vi "Initialize Picture Drag.vi"(6 "wheel index":i32, 8 "error in (no error)":errorcluster, 9 "dragging mode":T1, 10 "global mouse position":cluster{"x":dbl, "y":dbl}, 11 "dialog info in":T2={"steering frame ref"=refnum, "active wheel indexes"=[], "FP Refs"={"VI Refnum"=refnum, "Menu Ref"=refnum, "Sub Panel"=refnum, "picture"=refnum, "Steering Type"=refnum, "zoom in"=refnum, "zoom out"=refnum, "zoom extents"=refnum, "Wheels"=refnum, "Add Wheel"=refnum, "Remove Wheel"=refnum, "Copy Wheel"=refnum, "Angle Units"=refnum}, "subpanel info"={"subpanel VI refs"=[], "subpanel types"=[], "main to subpanel command events"=[]}, "picture dragging state"={"dragging"=FALSE, "wheel index"=-1, "dragging mode"=enum."translate", "wheel start position"={"x"=0.0, "y"=0.0, "theta"=0.0}, "relative mouse position"={"x"=0.0, "y"=0.0}, "relative mouse init angle (rad)"=0.0}, "picture size (pixels)"={"Width"=500, "Height"=500}, "picture grid"=bytes[0], "click zones group"={"click zones array"=[], "num click zones"=0}, "draw options"={"draw wheel states?"=FALSE, "highlight wheel index"=-1, "pixels per unit"=10.0, "draw forward velocity?"=FALSE, "velocity scale"=1.0}}) -> (0 "error out":errorcluster, 3 "dialog info out":T2={"steering frame ref"=refnum, "active wheel indexes"=[], "FP Refs"={"VI Refnum"=refnum, "Menu Ref"=refnum, "Sub Panel"=refnum, "picture"=refnum, "Steering Type"=refnum, "zoom in"=refnum, "zoom out"=refnum, "zoom extents"=refnum, "Wheels"=refnum, "Add Wheel"=refnum, "Remove Wheel"=refnum, "Copy Wheel"=refnum, "Angle Units"=refnum}, "subpanel info"={"subpanel VI refs"=[], "subpanel types"=[], "main to subpanel command events"=[]}, "picture dragging state"={"dragging"=FALSE, "wheel index"=-1, "dragging mode"=enum."translate", "wheel start position"={"x"=0.0, "y"=0.0, "theta"=0.0}, "relative mouse position"={"x"=0.0, "y"=0.0}, "relative mouse init angle (rad)"=0.0}, "picture size (pixels)"={"Width"=500, "Height"=500}, "picture grid"=bytes[0], "click zones group"={"click zones array"=[], "num click zones"=0}, "draw options"={"draw wheel states?"=FALSE, "highlight wheel index"=-1, "pixels per unit"=10.0, "draw forward velocity?"=FALSE, "velocity scale"=1.0}})   [LabVIEW 2017, in "NI_Robotics_Configure Steering Frame.lvlib"]
uses:
  <vilib>/robotics/Dialog/Configure Steering Frame/NI_Robotics_Configure Steering Frame.lvlib
  <vilib>/robotics/Dialog/Configure Steering Frame/Dialog Info.ctl
  <vilib>/robotics/Steering/Steering Frame/NI_Robotics_Steering Frame.lvclass
  <vilib>/robotics/Dialog/Configure Steering Frame/FP Refs.ctl
  <vilib>/robotics/Dialog/Configure Steering Frame/Subpanel Info.ctl
  <vilib>/robotics/Dialog/Configure Steering Frame/Main to Subpanel Command Event.ctl
  <vilib>/robotics/Dialog/Configure Steering Frame/Main to Subpanel Command.ctl
  <vilib>/robotics/Dialog/Configure Steering Frame/Dragging State.ctl
  <vilib>/robotics/Dialog/Configure Steering Frame/Dragging Mode.ctl
  <vilib>/Utility/miscctls.llb/LVBoundsTypeDef.ctl
  <vilib>/robotics/Dialog/Configure Steering Frame/Click Zone.ctl
  <vilib>/robotics/Utilities/Visualization/Steering Visualization/Steering Picture/Draw Steering Frame Options.ctl
  <vilib>/robotics/Steering/Steering Frame/NI_Robotics_Steering Frame.lvclass/NI_Robotics_Steering Frame.ctl
  <vilib>/Analysis/coordinate.llb/Angle Rotation (scalar).vi
  <vilib>/robotics/Steering/Steering Frame/Get Multiple Wheels in Steering Frame.vi
  <vilib>/Analysis/coordinate.llb/Wrap Angle (scalar).vi
  <vilib>/robotics/Steering/Wheel/NI_Robotics_Wheel.lvclass
  <vilib>/Analysis/NI_AAL_Angle.lvlib
  <vilib>/robotics/Utilities/Visualization/Steering Visualization/Steering Picture/NI_Robotics_Steering Picture.lvlib
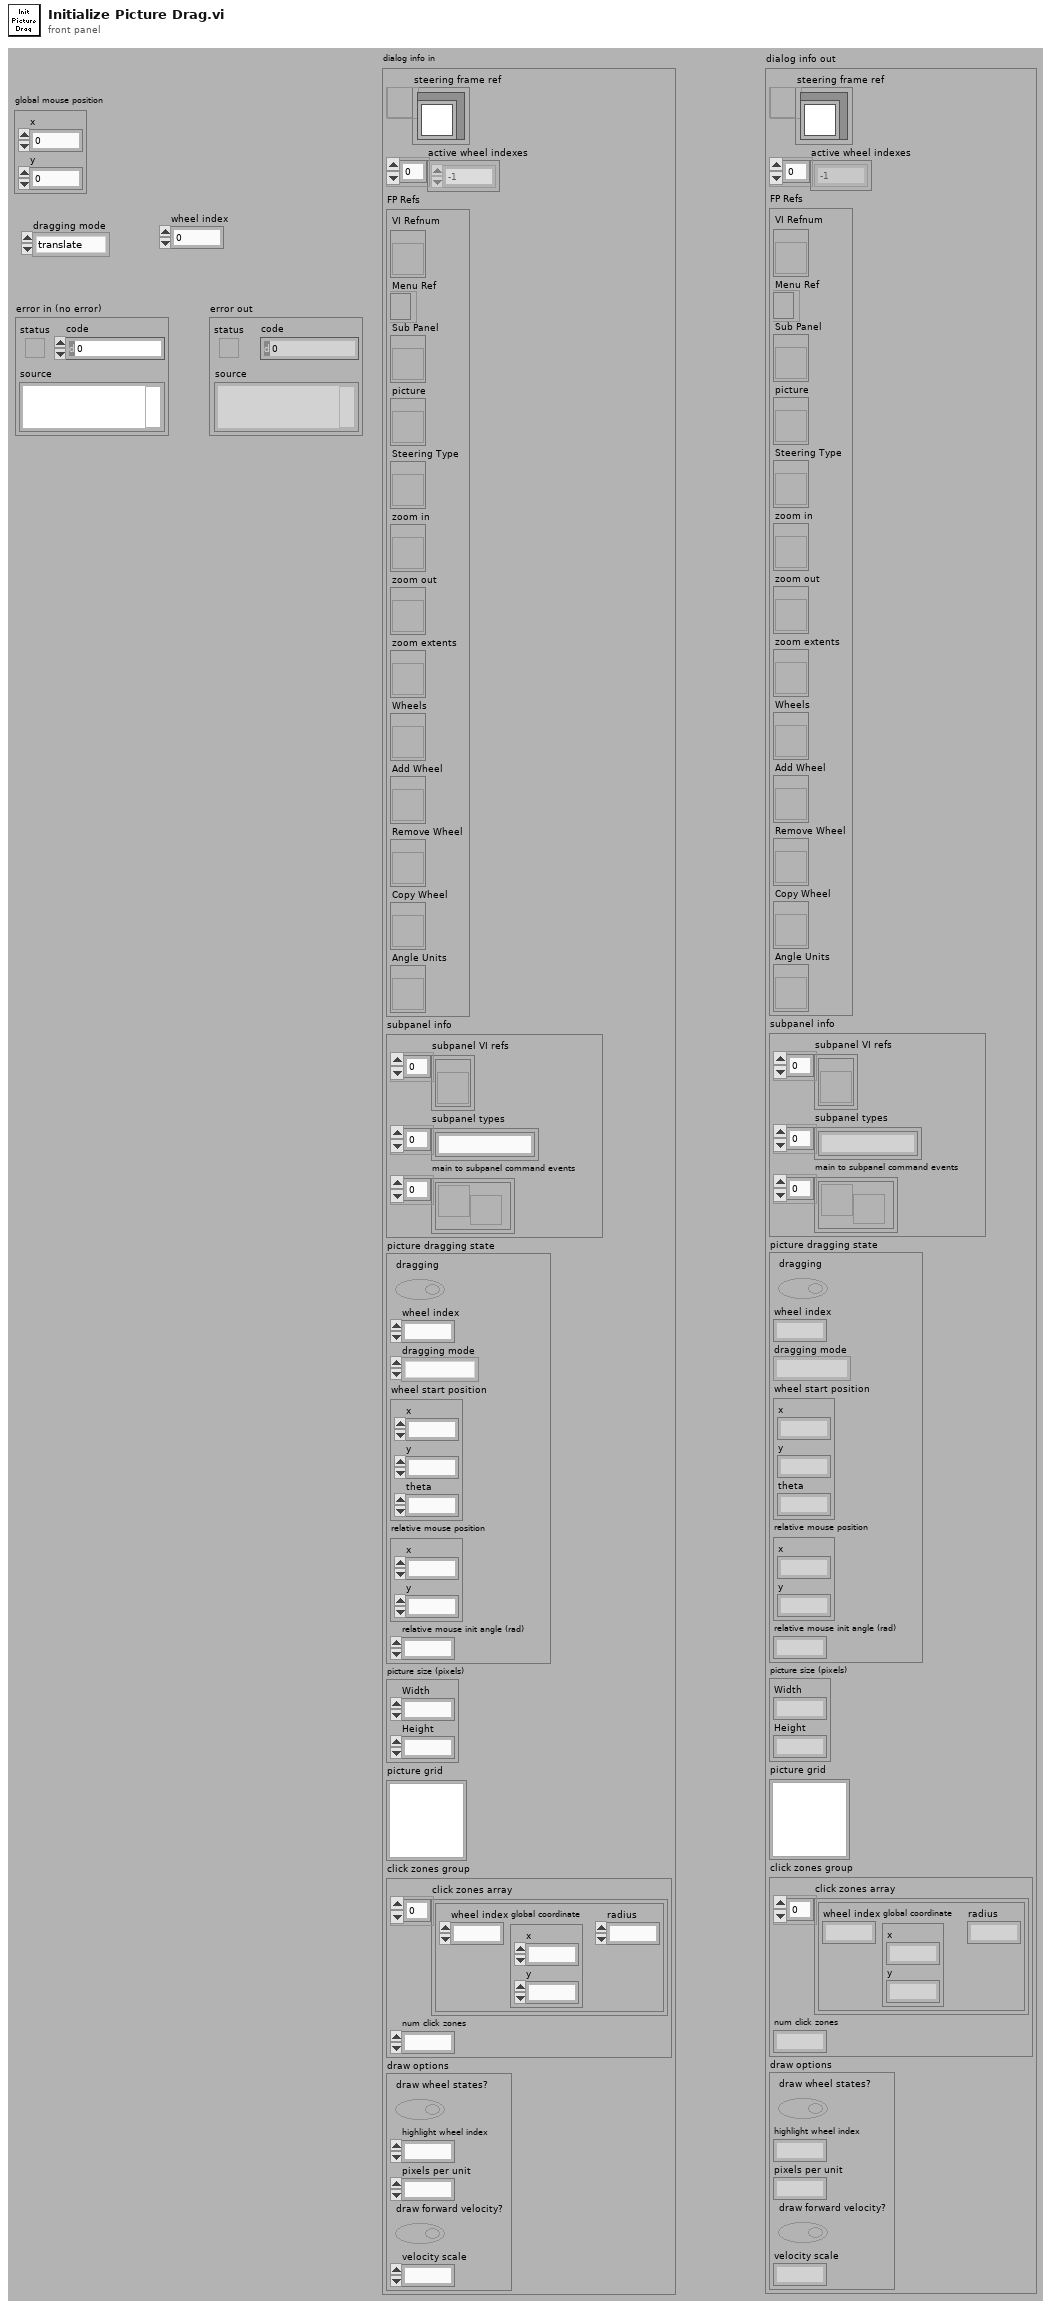
[diagram p1: front panel]
types:
  T1 = typedef "NI_Robotics_Configure Steering Frame.lvlib/Dragging Mode.ctl" = enum16{"translate", "rotate"}
  T2 = typedef "NI_Robotics_Configure Steering Frame.lvlib/Dialog Info.ctl" = cluster{"steering frame ref":refnum<data-value>, "active wheel indexes":i32[], "FP Refs":T3, "subpanel info":T4, "picture dragging state":T6, "picture size (pixels)":T7, "picture grid":picture, "click zones group":cluster{"click zones array":T8[], "num click zones":i32}, "draw options":T9}
  T3 = typedef "NI_Robotics_Configure Steering Frame.lvlib/FP Refs.ctl" = cluster{"VI Refnum":refnum<vi>, "Menu Ref":refnum<k9>, "Sub Panel":refnum<vi>, "picture":refnum<vi>, "Steering Type":refnum<vi>, "zoom in":refnum<vi>, "zoom out":refnum<vi>, "zoom extents":refnum<vi>, "Wheels":refnum<vi>, "Add Wheel":refnum<vi>, "Remove Wheel":refnum<vi>, "Copy Wheel":refnum<vi>, "Angle Units":refnum<vi>}
  T4 = typedef "NI_Robotics_Configure Steering Frame.lvlib/Subpanel Info.ctl" = cluster{"subpanel VI refs":refnum<vi>[], "subpanel types":string[], "main to subpanel command events":T5[]}
  T5 = typedef "NI_Robotics_Configure Steering Frame.lvlib/Main to Subpanel Command Event.ctl" = refnum<user-event>
  T6 = typedef "NI_Robotics_Configure Steering Frame.lvlib/Dragging State.ctl" = cluster{"dragging":bool, "wheel index":i32, "dragging mode":T1, "wheel start position":cluster{"x":dbl, "y":dbl, "theta":dbl}, "relative mouse position":cluster{"x":dbl, "y":dbl}, "relative mouse init angle (rad)":dbl}
  T7 = typedef "LVBoundsTypeDef.ctl" = cluster{"Width":u32, "Height":u32}
  T8 = typedef "NI_Robotics_Configure Steering Frame.lvlib/Click Zone.ctl" = cluster{"wheel index":i32, "global coordinate":cluster{"x":dbl, "y":dbl}, "radius":dbl}
  T9 = typedef "NI_Robotics_Steering Picture.lvlib/Draw Steering Frame Options.ctl" = cluster{"draw wheel states?":bool, "highlight wheel index":i32, "pixels per unit":dbl, "draw forward velocity?":bool, "velocity scale":dbl}
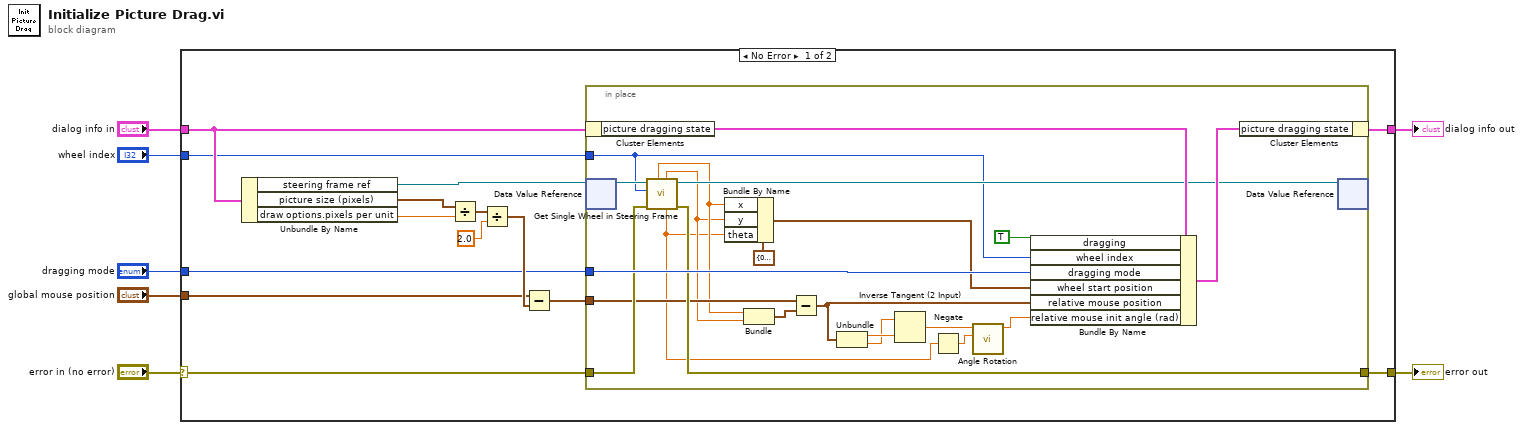
[diagram p0: block diagram]
diagram:
  n1 = case shown="No Error" "error in (no error)" {
    selector: "error in (no error)" -> [w12 w45]
    tunnel: "dialog info in" -> [w17 w44]
    tunnel: [w10 w45] -> w5
    tunnel: [w16 w44] -> w4
    tunnel: "global mouse position" -> [w18 _]
    tunnel: "dragging mode" -> [w13 _]
    tunnel: "wheel index" -> [w8 _]
    frame No Error {
      n2 = Unbundle By Name(w17) -> ("steering frame ref"=w15:refnum<data-value>, "picture size (pixels)"=w20:T7, "draw options.pixels per unit"=w9:dbl)
      n3 = Divide(x=w20, y=w9) -> (x/y=w21:cluster{"Width":dbl, "Height":dbl})
      n4 = Divide(x=w21, y=2.0) -> (x/y=w19:cluster{"Width":dbl, "Height":dbl})
      n5 = Subtract(x=w18, y=w19) -> (x-y=w14:cluster{dbl, dbl})
      n6 = in-place {
        in-place-border: w8 -> [w37]
        in-place-border: w13 -> [w40]
        in-place-border: w14 -> [w33]
        in-place-border: w12 -> [w35]
        in-place-border: [w34] -> w10
        n7 = in-place-cluster #1(w17) -> ("picture dragging state"=w43:T6)
        n8 = in-place-dvr #2(w15) -> (w39:refnum<class "NI_Robotics_Steering Frame.lvclass">)  [unwired: 1 out]
        n9 = call <vilib>:"Get Single Wheel in Steering Frame.vi"("error in (no error)"=w35, "wheel index"=w37, "steering frame in"=w39) -> ("error out"=w34:errorcluster, "steering frame out"=w38:refnum<class "NI_Robotics_Steering Frame.lvclass">, "frame angle (rad)"=w25:dbl, "y position"=w30:dbl, "x position"=w31:dbl)  [unwired: 2 in, 2 out]
        n10 = Bundle By Name(cluster=cluster{"x":dbl, "y":dbl, "theta":dbl} {"x"=0.0, "y"=0.0, "theta"=0.0} ("wheel start position"), "x"=w31, "y"=w30, "theta"=w25) -> (w32:cluster{"x":dbl, "y":dbl, "theta":dbl})
        n11 = Bundle("x position"=w31, "y position"=w30) -> (w27:cluster{"x position":dbl, "y position":dbl})  [unwired: 1 in]
        n12 = Subtract(x=w33, y=w27) -> (x-y=w26:cluster{dbl, dbl})
        n13 = Unbundle(w26) -> (w29:dbl, w28:dbl)
        n14 = Inverse Tangent (2 Input)(1:w29, 2:w28) -> (0:w24:dbl)
        n15 = Negate(x=w25) -> (-x=w23:dbl)
        n16 = call-poly <vilib>:"Angle Rotation.vi"("counterclockwise rotation"=w23, "angle"=w24) -> ("rotated angle"=w22:dbl)  [unwired: 8 in, 1 out]
        n17 = Bundle By Name(cluster=w43, "dragging"=TRUE, "wheel index"=w37, "dragging mode"=w40, "wheel start position"=w32, "relative mouse position"=w26, "relative mouse init angle (rad)"=w22) -> (w42:T6)
        n18 = in-place-cluster #1("picture dragging state"=w42) -> (w16:T2)
        n19 = in-place-dvr #2(w38) -> ()  [unwired: 2 out]
      }
    }
    frame Error {
    }
  }
  "dialog info out" <- w4
  "error out" <- w5
